vi "iow28_io-ports_read.vi"() -> ()   [LabVIEW 2011]
panel:
  in  "Stopp":bool
  out "arrayout":u8[](array[numeric]) format="%x"
  out "Error Read":errorcluster caption="error"
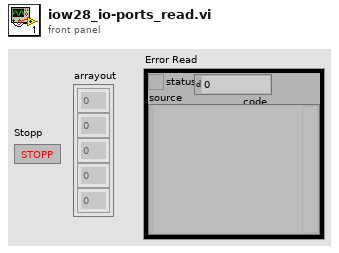
[diagram p1: front panel]
types:
  T1 = typedef "IOWarrior_Handle.ctl" = cluster{"Handle":u32, "Serial Number":string, "type of Warrior":T2, "Root Handle":bool, "Revision":u16}
  T2 = typedef "IOWarrior_Type.ctl" = enum16{"invalid", "IOW24", "IOW40", "IOW56", "IOPV1", "IOPV2", "IOW28"}
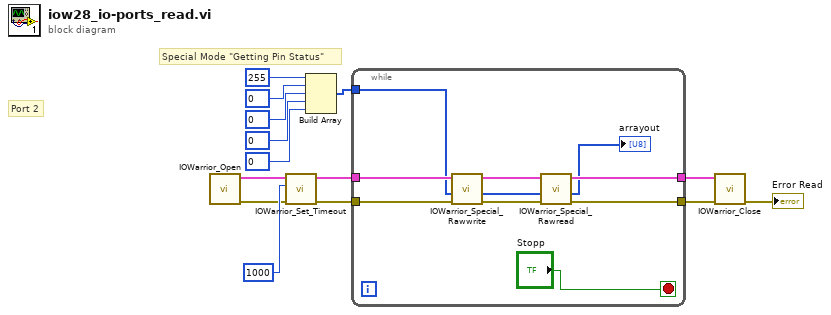
[diagram p0: block diagram]
diagram:
  # "Port 2"
  # "Special Mode \"Getting Pin Status\""
  n1 = call "IOWarrior_Open.vi"() -> ("err out"=w12:errorcluster, "IOWarriorHandle"=w13:T1)  [unwired: 9 in, 1 out]
  n2 = call "IOWarrior_Set_Timeout.vi"("err in"=w12, "timeout_ms(1000)"=1000, "devHandle"=w13) -> ("err out"=w10:errorcluster, "devHandleout"=w11:T1)  [unwired: 6 in, 1 out]
  n3 = Build Array(u8 255, u8 0, u8 0, u8 0, u8 0) -> (w5:u8[])
  n4 = while {
    tunnel: w11 -> [w20]
    tunnel: w10 -> [w21]
    tunnel: [w24] -> w9
    tunnel: [w23] -> w8
    tunnel: w5 -> [w16]
    stop <- "Stopp" stop-if-true
    n5 = call "IOWarrior_Special_Rawwrite.vi"("err in"=w21, "Array_in"=w16, "devHandle"=w20) -> ("err out"=w18:errorcluster, "array_out"=w17:u8[], "devHandleout"=w19:T1)  [unwired: 6 in]
    n6 = call "IOWarrior_Special_Rawread.vi"("err in"=w18, "array"=w17, "devHandle"=w19) -> ("err out"=w24:errorcluster, "arrayout"=→"arrayout":u8[], "devHandleout"=w23:T1)  [unwired: 6 in]
  }
  n7 = call "IOWarrior_Close.vi"("err in"=w9, "devHandle"=w8) -> ("err out"=→"Error Read":errorcluster)  [unwired: 8 in, 1 out]
